vi "nanocal_process tdms file.vi"(7 "actions":T1, 8 "Error In":errorcluster, 9 "Configuration":T2={"New start time"=nan, "New end time"=nan, "Output file format"=enum."ASCII", "Save ASCII column names"=TRUE, "Prepend binary array size"=FALSE, "buffer size (-1: all)"=100000, "Group"="p", "New dt"=nan, "IGORify column names"=TRUE, "eliminate spaces in col name"=TRUE, "Channels"=["jsdhgv", "lsjdfh", "ajlsd"]} {"buffer size (-1: all)" format="%.0p"; "New start time" format="%#_10p"}, 11 "tdms file IN":path=path "/Users/arkadyshekhter/Library/CloudStorage/Dropbox/desktop_data/nanocal-cell12-Mar2020/March_2020/032620/m004_032620.tdms") -> (0 "Error Out":errorcluster, 1 "new Configuration":T2={"New start time"=nan, "New end time"=nan, "Output file format"=enum."ASCII", "Save ASCII column names"=TRUE, "Prepend binary array size"=FALSE, "buffer size (-1: all)"=100000, "Group"="p", "New dt"=nan, "IGORify column names"=TRUE, "eliminate spaces in col name"=TRUE, "Channels"=["Time", "frequency (Hz)", "Cs/T (J/K^2)", "Ts (K)", "Ts^2 (K^2)", "Tr (K)", "Cs (J/K)", "Cr (J/K)", "Ks (W/K)", "Kr (W/K)", "Rs-therm (Ohm)", "Rr-therm (Ohm)", "Cr/T (J/K^2)", "dlogR/dlogT -- S  (a.u.)", "tau (s)", "tan(phi) (a.u)", "Ts,ac (K)", "Tr,ac (K)", "Hs,ac,out (V)", "Offset,dc,out (V)", "Vdiff,ac (V)", "Vdiff,ac,phase (deg)", "Stherm,ac,out (V)", "Rtherm,ac,out (V)", "CV1 -- Re (V)", "CV1 -- Im (V)", "DV2 -- Re (V)", "DV2 -- Im (V)", "AV2 -- Re (V)", "AV2 -- Im (V)", "Vdiff,norm, Re (V)", "Vdiff,norm, Im (V)", "LakeShore 336 (12) A", "LakeShore 336 (12) B", "LakeShore 336 (12) C", "LakeShore 336 (12) D", "pos", "field (T)"]} {"buffer size (-1: all)" format="%.0p"; "New start time" format="%#_10p"}, 2 "dat file out":path=path "/Users/arkadyshekhter/Library/CloudStorage/Dropbox/desktop_data/nanocal-cell12-Mar2020/March_2020/032620/m004_032620.dat", 3 "tdms file OUT":path=path "/Users/arkadyshekhter/Library/CloudStorage/Dropbox/desktop_data/nanocal-cell12-Mar2020/March_2020/032620/m004_032620.tdms", 4 "ALL channel names":string[](array[string])=["Time", "frequency (Hz)", "Cs/T (J/K^2)", "Ts (K)", "Ts^2 (K^2)", "Tr (K)", "Cs (J/K)", "Cr (J/K)", "Ks (W/K)", "Kr (W/K)", "Rs-therm (Ohm)", "Rr-therm (Ohm)", "Cr/T (J/K^2)", "dlogR/dlogT -- S  (a.u.)", "tau (s)", "tan(phi) (a.u)", "Ts,ac (K)", "Tr,ac (K)", "Hs,ac,out (V)", "Offset,dc,out (V)", "Vdiff,ac (V)", "Vdiff,ac,phase (deg)", "Stherm,ac,out (V)", "Rtherm,ac,out (V)", "CV1 -- Re (V)", "CV1 -- Im (V)", "DV2 -- Re (V)", "DV2 -- Im (V)", "AV2 -- Re (V)", "AV2 -- Im (V)", "Vdiff,norm, Re (V)", "Vdiff,norm, Im (V)", "LakeShore 336 (12) A", "LakeShore 336 (12) B", "LakeShore 336 (12) C", "LakeShore 336 (12) D", "pos", "field (T)"])   [LabVIEW 2021]
uses:
  NHMFL_Core/Libraries/File/File Format Converter/Format Converter Configuration.ctl
  nanocal_raw_file_manage_fieldname_V1.ctl
  nanocal_process_tdms_file_control.ctl
  <vilib>/Utility/TDMS File Viewer/NI_TDMS File Viewer.lvlib
  string array manage control.ctl
panel:
  out "header OUT":string
  out "Map of column induices":map{T3, i32}(c390)
  in  "header IN":string
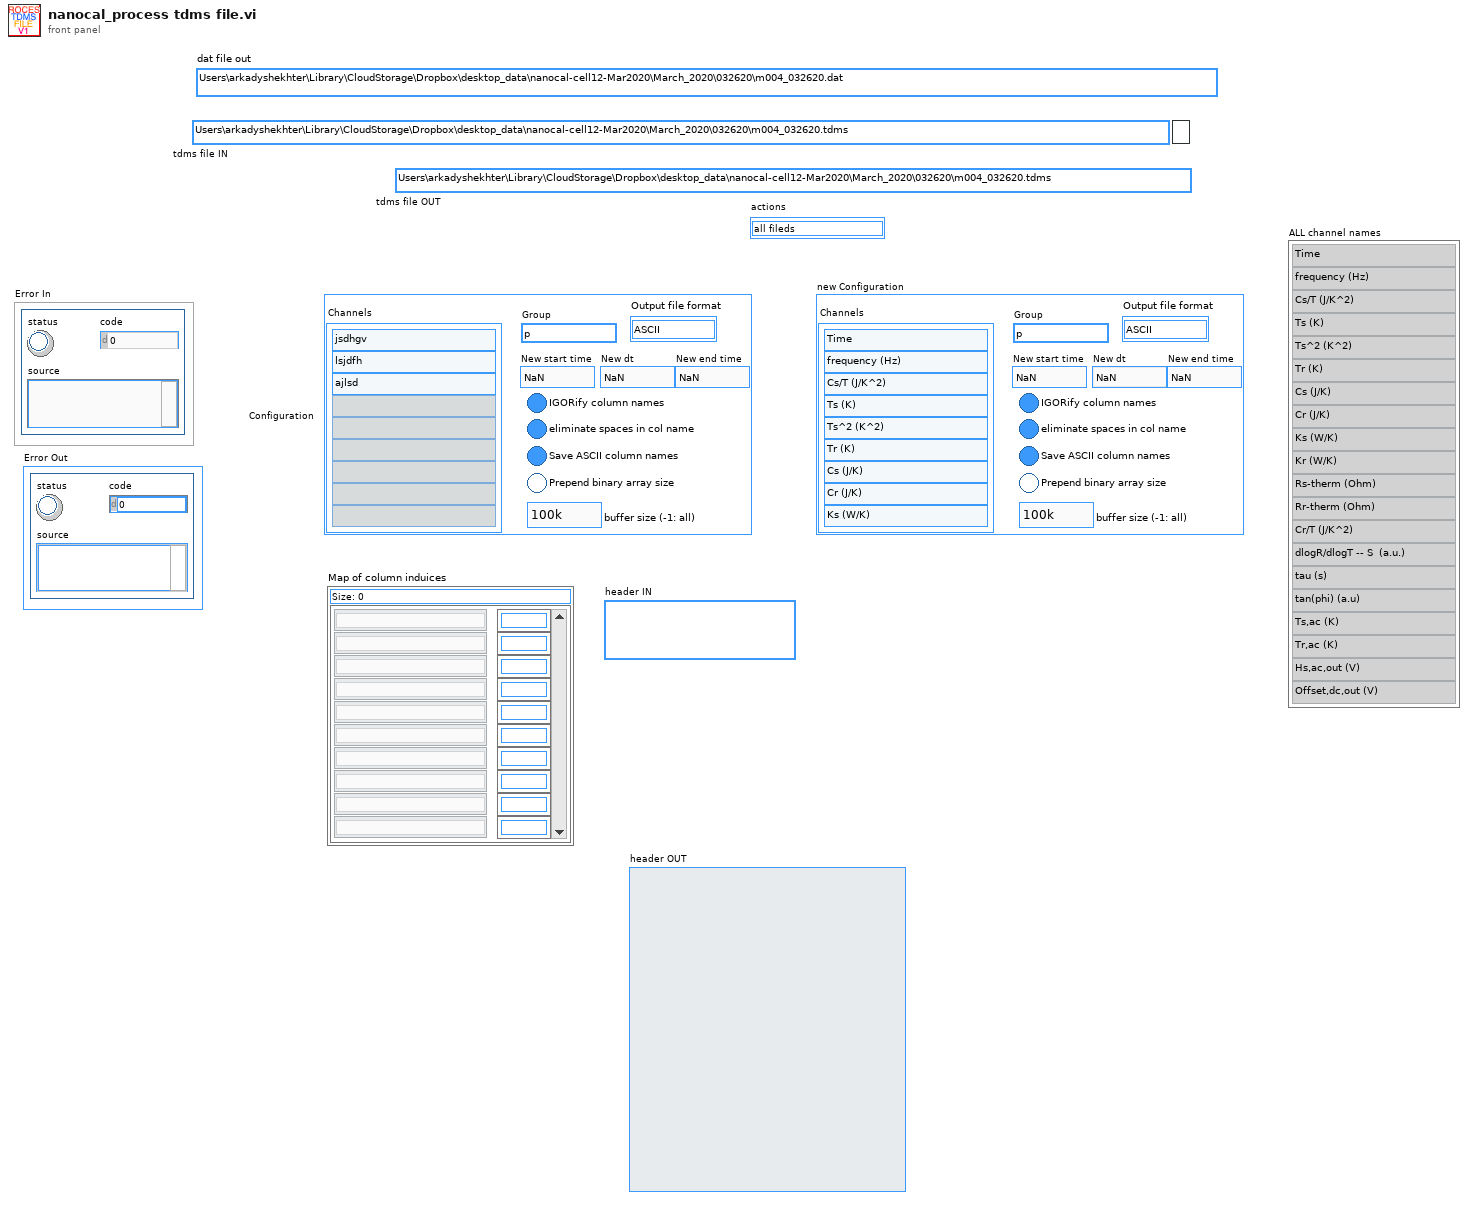
[diagram p1: front panel]
types:
  T1 = typedef "nanocal_process_tdms_file_control.ctl" = enum16{"all fileds", "subset of fields"}
  T2 = typedef "Format Converter Configuration.ctl" = cluster{"New start time":dbl, "New end time":dbl, "Output file format":enum16{"ASCII", "BINARY", "TDMS"}, "Save ASCII column names":bool, "Prepend binary array size":bool, "buffer size (-1: all)":i64, "Group":string, "New dt":dbl, "IGORify column names":bool, "eliminate spaces in col name":bool, "Channels":string[]}
  T3 = typedef "nanocal_raw_file_manage_fieldname_V1.ctl" = enum16{"f (Hz)", "S phase (deg)", "R phase (deg)", "Ts,ac (K)", "Tr,ac (K)", "PHs (W)", "PHr (W)", "Time (s)", "Tdiff,ac (K)", "Ts (K)", "Tr (K)", "|dlnR/dlnT| S", "|dlnR/dlnT| R", "Rs (ohm)", "Rr (ohm)"}
  T4 = typedef "string array manage control.ctl" = enum16{"intersection", "match pattern"}
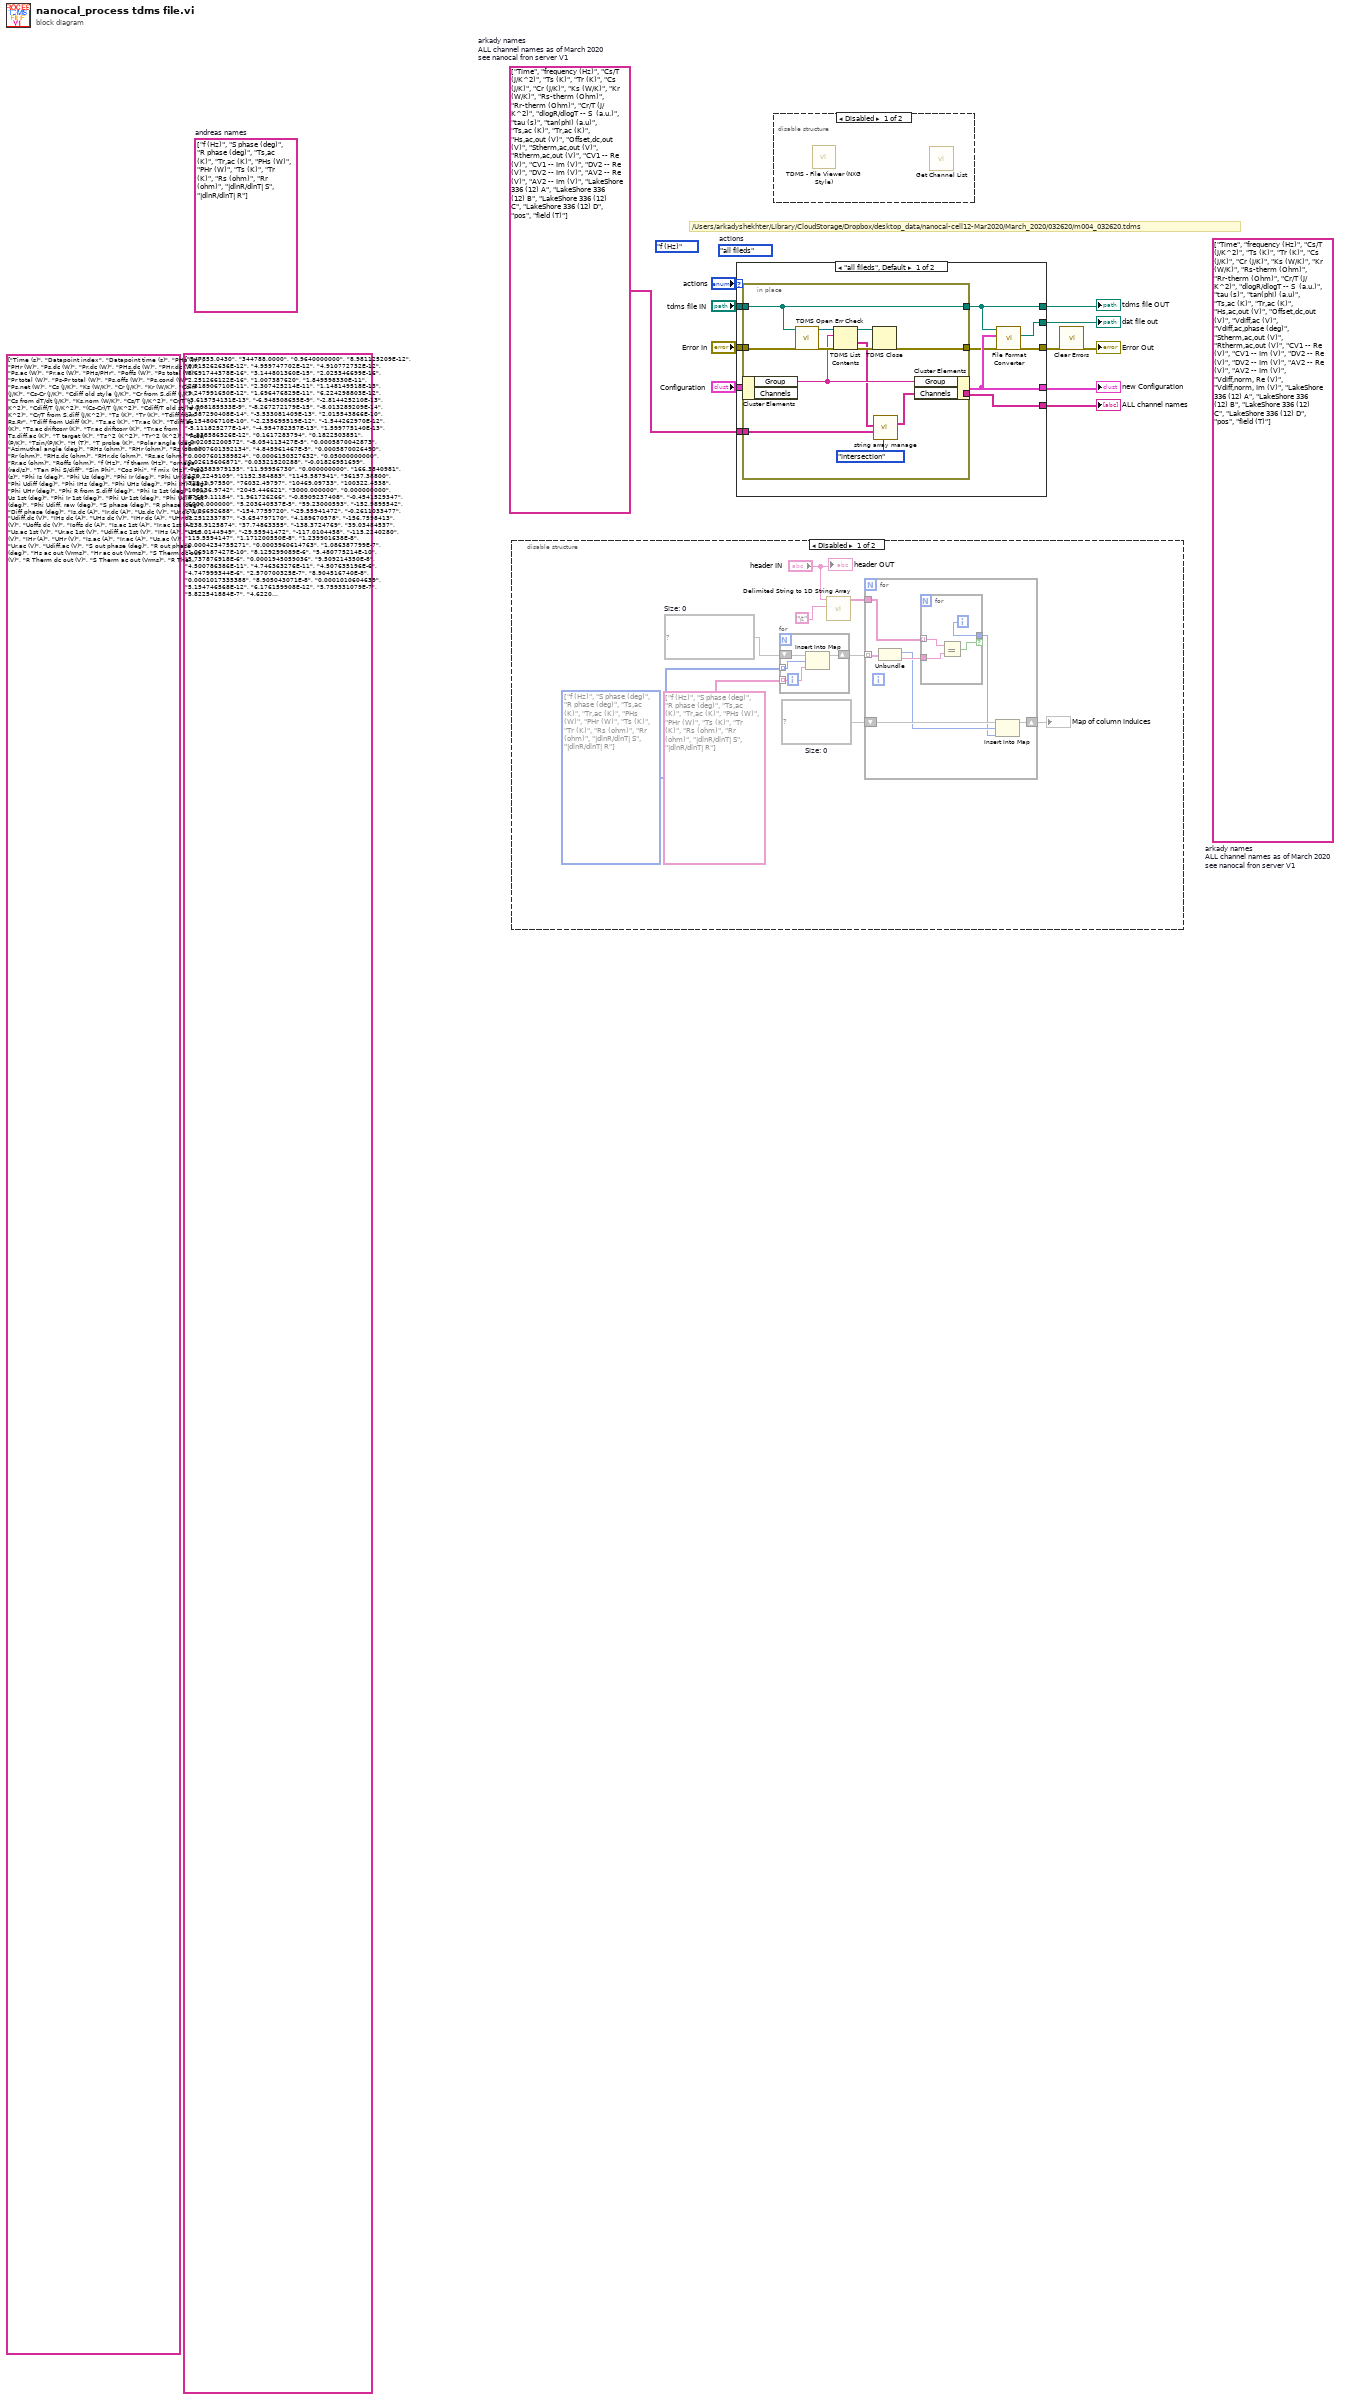
[diagram p0: block diagram]
diagram:
  w1 = string[] ["Time", "frequency (Hz)", "Cs/T (J/K^2)", "Ts (K)", "Tr (K)", "Cs (J/K)", "Cr (J/K)", "Ks (W/K)", "Kr (W/K)", "Rs-therm (Ohm)", "Rr-therm (Ohm)", "Cr/T (J/K^2)", "dlogR/dlogT -- S  (a.u.)", "tau (s)", "tan(phi) (a.u)", "Ts,ac (K)", "Tr,ac (K)", "Hs,ac,out (V)", "Offset,dc,out (V)", "Stherm,ac,out (V)", "Rtherm,ac,out (V)", "CV1 -- Re (V)", "CV1 -- Im (V)", "DV2 -- Re (V)", "DV2 -- Im (V)", "AV2 -- Re (V)", "AV2 -- Im (V)", "LakeShore 336 (12) A", "LakeShore 336 (12) B", "LakeShore 336 (12) C", "LakeShore 336 (12) D", "pos", "field (T)"]  # arkady names ALL channel names as of March 2020 see nanocal fron server V1
  (unwired) nanocal_process_tdms_file_control."all fileds"  # actions
  (unwired) nanocal_raw_file_manage_fieldname_V1."f (Hz)" ("field names")
  (unwired) string[] ["Time", "frequency (Hz)", "Cs/T (J/K^2)", "Ts (K)", "Tr (K)", "Cs (J/K)", "Cr (J/K)", "Ks (W/K)", "Kr (W/K)", "Rs-therm (Ohm)", "Rr-therm (Ohm)", "Cr/T (J/K^2)", "dlogR/dlogT -- S  (a.u.)", "tau (s)", "tan(phi) (a.u)", "Ts,ac (K)", "Tr,ac (K)", "Hs,ac,out (V)", "Offset,dc,out (V)", "Vdiff,ac (V)", "Vdiff,ac,phase (deg)", "Stherm,ac,out (V)", "Rtherm,ac,out (V)", "CV1 -- Re (V)", "CV1 -- Im (V)", "DV2 -- Re (V)", "DV2 -- Im (V)", "AV2 -- Re (V)", "AV2 -- Im (V)", "Vdiff,norm, Re (V)", "Vdiff,norm, Im (V)", "LakeShore 336 (12) A", "LakeShore 336 (12) B", "LakeShore 336 (12) C", "LakeShore 336 (12) D", "pos", "field (T)"]  # arkady names ALL channel names as of March 2020 see nanocal fron server V1
  (unwired) string[] ["f (Hz)", "S phase (deg)", "R phase (deg)", "Ts,ac (K)", "Tr,ac (K)", "PHs (W)", "PHr (W)", "Ts (K)", "Tr (K)", "Rs (ohm)", "Rr (ohm)", "|dlnR/dlnT| S", "|dlnR/dlnT| R"]  # andreas names
  (unwired) string[] ["547853.0430", "344788.0000", "0.9640000000", "8.981125209E-12", "8.915262636E-12", "4.959747702E-12", "4.910772732E-12", "8.691744378E-16", "3.144801360E-15", "2.025346699E-16", "2.251266122E-16", "1.007387620", "1.849598330E-11", "2.318906710E-11", "2.307425214E-11", "1.148149518E-13", "9.247991650E-12", "1.696476829E-11", "6.224298803E-12", "-3.615754131E-13", "-6.948508655E-9", "-2.814425210E-13", "-4.998185533E-9", "-8.267272179E-15", "-8.013289209E-14", "2.587290408E-14", "-3.533081409E-13", "2.015543866E-10", "6.154806710E-10", "-2.235695519E-12", "-1.544262970E-12", "-5.111825277E-14", "-4.954782357E-13", "1.599775140E-13", "-1.938586526E-12", "0.1617283794", "0.1822503851", "-0.02052200572", "-8.054113427E-5", "0.0005870042873", "0.0007601392134", "4.845961467E-5", "0.0005870026490", "0.0007601389824", "0.0006150327632", "0.05000000000", "0.02615606871", "0.03321520288", "-0.01826951699", "-0.03583979135", "11.99956730", "0.000000000", "166.3840981", "120.2249109", "1152.384883", "1145.587941", "36157.38800", "31942.97550", "76032.49797", "10469.09733", "100322.4538", "100136.9742", "2045.446621", "3000.000000", "0.000000000", "37699.11184", "1.961726266", "-0.8909237408", "-0.4541529347", "6000.000000", "5.203640537E-5", "59.23000593", "-152.9895542", "71.26692688", "-154.7759720", "-29.55941472", "-0.2611033477", "7.251233787", "-3.654797170", "4.189670578", "-156.7598413", "-138.9125874", "37.74863355", "-138.3724769", "39.03484537", "-115.0144949", "-29.55941472", "-117.0104458", "-115.2240280", "119.5594147", "1.171200550E-8", "1.239901638E-8", "0.0004234755271", "0.0003960614763", "1.086387799E-7", "1.069187427E-10", "8.129299089E-6", "5.480775214E-10", "5.737876918E-6", "0.0001945059036", "9.509214350E-8", "4.500786386E-11", "4.746363276E-11", "4.507635196E-6", "4.747999344E-6", "2.570700325E-7", "8.904516740E-8", "0.0001017335388", "8.905043071E-8", "0.0001010604639", "5.154746568E-12", "6.176159908E-12", "5.759331079E-7", "5.822541884E-7", "4.622022938E-8", "0.000000000", "0.000000000", "0.009030217479", "0.009030217479", "0.001382604241", "0.001487392001", "0.000000000", "0.000000000", "0.009530331008", "0.000000000", "0.000000000", "0.000000000", "1.361573880", "3.765686503", "36157.38800", "31942.97550", "-18107.21790", "-11982.49189", "0.7014008160", "0.6673683771", "0.03088148519", "0.004354902059", "1.234560000"] ("string array")
  (unwired) string[] ["Time (s)", "Datapoint index", "Datapoint time (s)", "PHs (W)", "PHr (W)", "Ps,dc (W)", "Pr,dc (W)", "PHs,dc (W)", "PHr,dc (W)", "Ps,ac (W)", "Pr,ac (W)", "PHs/PHr", "Poffs (W)", "Ps total (W)", "Pr total (W)", "Ps-Pr total (W)", "Ps,offs (W)", "Ps,cond (W)", "Ps,net (W)", "Cs (J/K)", "Ks (W/K)", "Cr (J/K)", "Kr (W/K)", "Cdiff (J/K)", "Cs-Cr (J/K)", "Cdiff old style (J/K)", "Cr from S,diff (J/K)", "Cs from dT/dt (J/K)", "Ks,nom (W/K)", "Cs/T (J/K^2)", "Cr/T (J/K^2)", "Cdiff/T (J/K^2)", "(Cs-Cr)/T (J/K^2)", "Cdiff/T old style (J/K^2)", "Cr/T from S,diff (J/K^2)", "Ts (K)", "Tr (K)", "Tdiff from Rs,Rr", "Tdiff from Udiff (K)", "Ts,ac (K)", "Tr,ac (K)", "Tdiff,ac (K)", "Ts,ac driftcorr (K)", "Tr,ac driftcorr (K)", "Tr,ac from Ts,diff,ac (K)", "T target (K)", "Ts^2 (K^2)", "Tr^2 (K^2)", "Tcos/(P/K)", "Tsin/(P/K)", "H (T)", "T probe (K)", "Polar angle (deg)", "Azimuthal angle (deg)", "RHs (ohm)", "RHr (ohm)", "Rs (ohm)", "Rr (ohm)", "RHs,dc (ohm)", "RHr,dc (ohm)", "Rs,ac (ohm)", "Rr,ac (ohm)", "Roffs (ohm)", "f (Hz)", "f therm (Hz)", "omega (rad/s)", "Tan Phi S/diff", "Sin Phi", "Cos Phi", "f mix (Hz)", "tau (s)", "Phi Is (deg)", "Phi Us (deg)", "Phi Ir (deg)", "Phi Ur (deg)", "Phi Udiff (deg)", "Phi IHs (deg)", "Phi UHs (deg)", "Phi IHr (deg)", "Phi UHr (deg)", "Phi R from S,diff (deg)", "Phi Is 1st (deg)", "Phi Us 1st (deg)", "Phi Ir 1st (deg)", "Phi Ur 1st (deg)", "Phi Udiff 1st (deg)", "Phi Udiff, raw (deg)", "S phase (deg)", "R phase (deg)", "Diff phase (deg)", "Is,dc (A)", "Ir,dc (A)", "Us,dc (V)", "Ur,dc (V)", "Udiff,dc (V)", "IHs dc (A)", "UHs dc (V)", "IHr dc (A)", "UHr dc (V)", "Uoffs dc (V)", "Ioffs dc (A)", "Is,ac 1st (A)", "Ir,ac 1st (A)", "Us,ac 1st (V)", "Ur,ac 1st (V)", "Udiff,ac 1st (V)", "IHs (A)", "UHs (V)", "IHr (A)", "UHr (V)", "Is,ac (A)", "Ir,ac (A)", "Us,ac (V)", "Ur,ac (V)", "Udiff,ac (V)", "S out phase (deg)", "R out phase (deg)", "Hs ac out (Vrms)", "Hr ac out (Vrms)", "S Therm dc out (V)", "R Therm dc out (V)", "S Therm ac out (Vrms)", "R Therm ac out (Vrms)", "Offset dc out (V)", "Hs dc out (V)", "Hr dc out (V)", "Offset ac out (Vrms)", "1+Rs/RIs factor", "1+RIs/Rs factor", "Rs,scaled (ohm)", "Rr,scaled (ohm)", "R lead S (ohm)", "R lead R (ohm)", "|dlnR/dlnT| S", "|dlnR/dlnT| R", "dTs/dt (mK/s)", "dTr/dt (mK/s)", "Test", ""] ("string array")
  # "/Users/arkadyshekhter/Library/CloudStorage/Dropbox/desktop_data/nanocal-cell12-Mar2020/March_2020/032620/m004_032620.tdms"
  n1 = disable-structure shown="Disabled" {
    frame Disabled {
      w16 = map{T3, i32} {}  # Size: 0
      w20 = map{T3, string} {}  # Size: 0
      w19 = T3[] [enum."f (Hz)", enum."S phase (deg)", enum."R phase (deg)", enum."Ts,ac (K)", enum."Tr,ac (K)", enum."PHs (W)", enum."PHr (W)", enum."Ts (K)", enum."Tr (K)", enum."Rs (ohm)", enum."Rr (ohm)", enum."|dlnR/dlnT| S", enum."|dlnR/dlnT| R"] items=["f (Hz)", "S phase (deg)", "R phase (deg)", "Ts,ac (K)", "Tr,ac (K)", "PHs (W)", "PHr (W)", "Time (s)", "Tdiff,ac (K)", "Ts (K)", "Tr (K)", "|dlnR/dlnT| S", "|dlnR/dlnT| R", "Rs (ohm)", "Rr (ohm)"]
      n2 = for {
        shift-right: [w34] -> w15
        shift-left: w20 -> [w35]
        tunnel: w19 -> [w33] mode=indexing
        tunnel: string[] ["f (Hz)", "S phase (deg)", "R phase (deg)", "Ts,ac (K)", "Tr,ac (K)", "PHs (W)", "PHr (W)", "Ts (K)", "Tr (K)", "Rs (ohm)", "Rr (ohm)", "|dlnR/dlnT| S", "|dlnR/dlnT| R"] -> [w32] mode=indexing
        n3 = Insert Into Map(map in=w35, key=w33, value=w32) -> (map out=w34:map{T3, string})  [unwired: 2 out]
      }
      n4 = call <vilib>:"Delimited String to 1D String Array.vi"("delimiter"="\t", "delimited string"="header IN") -> ("string array"=w14:string[])  [unwired: 9 in]
      n5 = for {
        shift-right: [w26] -> w12
        shift-left: w16 -> [w27]
        tunnel: w14 -> [w25]
        tunnel: w15 -> [w24] mode=indexing
        n6 = Unbundle(w24) -> ("field names"=w22:T3, w23:string)
        n7 = for {
          tunnel: w25 -> [w31] mode=indexing
          tunnel: w23 -> [w30]
          tunnel: [w29] -> w21 if=w28
          i -> [w29]
          n8 = Equal?(x=w31, y=w30) -> (x = y?=w28:bool)
        }
        n9 = Insert Into Map(map in=w27, key=w22, value=w21) -> (map out=w26:map{T3, i32})  [unwired: 2 out]
      }
      "Map of column induices" <- w12
      "header OUT" <- "header IN"
    }
    frame Enabled {
    }
  }
  n10 = case shown="\"all fileds\", Default" "actions" {
    tunnel: [w45 w59] -> w11
    tunnel: [w44 _] -> w10
    tunnel: "tdms file IN" -> [w40 w58]
    tunnel: "Configuration" -> [w43 w59]
    tunnel: "Error In" -> [w38 w60]
    tunnel: [w42 w60] -> w3
    tunnel: [w41 _] -> w6
    tunnel: [w39 w58] -> w4
    tunnel: w1 -> [w36 _]
    frame "all fileds", Default {
      n11 = in-place {
        in-place-border: [w47] -> w41
        in-place-border: w40 -> [w53]
        in-place-border: [w53] -> w39
        in-place-border: w38 -> [w52]
        in-place-border: [w51] -> w37
        in-place-border: w36 -> [w49]
        n12 = in-place-cluster #1(w43) -> ("Group"=w50:string)  [unwired: 1 out]
        n13 = call "TDMS Open Err Check.vi"("Error In"=w52, "File Path Control"=w53) -> ("Error Out"=w56:errorcluster, "tdms file out"=w57:refnum<k34>)  [unwired: 7 in, 1 out]
        n14 = TDMS List Contents(4:w56, 6:w50, 7:w57) -> (0:w54:errorcluster, 1:w48:string[], 3:w55:refnum<k34>)  [unwired: 1 out]
        n15 = TDMS Close(8:w54, 11:w55) -> (0:w51:errorcluster)  [unwired: 1 out]
        n16 = call "string array manage.vi"("actions"=string_array_manage_control."intersection", "Array 2 IN"=w49, "Array 1 IN"=w48) -> ("Array 1 OUT"=w47:string[])  [unwired: 7 in, 1 out]
        n17 = in-place-cluster #1("Group"=w50, "Channels"=w47) -> (w45:T2)
      }
      n18 = call "File Format Converter.vi"("Error In"=w37, "Configuration"=w45, "File"=w39) -> ("Error Out"=w42:errorcluster, "New file out"=w44:path)  [unwired: 6 in, 1 out]
    }
    frame "subset of fields" {
    }
  }
  "dat file out" <- w10
  "new Configuration" <- w11
  "ALL channel names" <- w6
  "tdms file OUT" <- w4
  n19 = disable-structure shown="Disabled" {
    frame Disabled {
      n20 = call <vilib>:"TDMS - File Viewer (NXG Style).vi"() -> ()  [unwired: 10 in, 2 out]
      n21 = call <vilib>:"Get Channel List.vi"() -> ()  [unwired: 5 in, 3 out]
    }
    frame Enabled {
    }
  }
  n22 = call <vilib>:"Clear Errors.vi"("error in (no error)"=w3) -> ("error out"=→"Error Out":errorcluster)  [unwired: 5 in, 1 out]
